vi "Forward Dynamics Demo.vi"() -> ()   [LabVIEW 2017, in "NI_Kinematics.lvlib"]
uses:
  <vilib>/robotics/Kinematics/NI_Kinematics.lvlib
panel:
  out "times":dbl[](array[numeric]) format="%#_40f"
  out "QD":dbl[][](array[numeric]) format="%#_6f"
  out "Q":dbl[][](array[numeric]) format="%#_6f"
  out "Time (ms)":u32
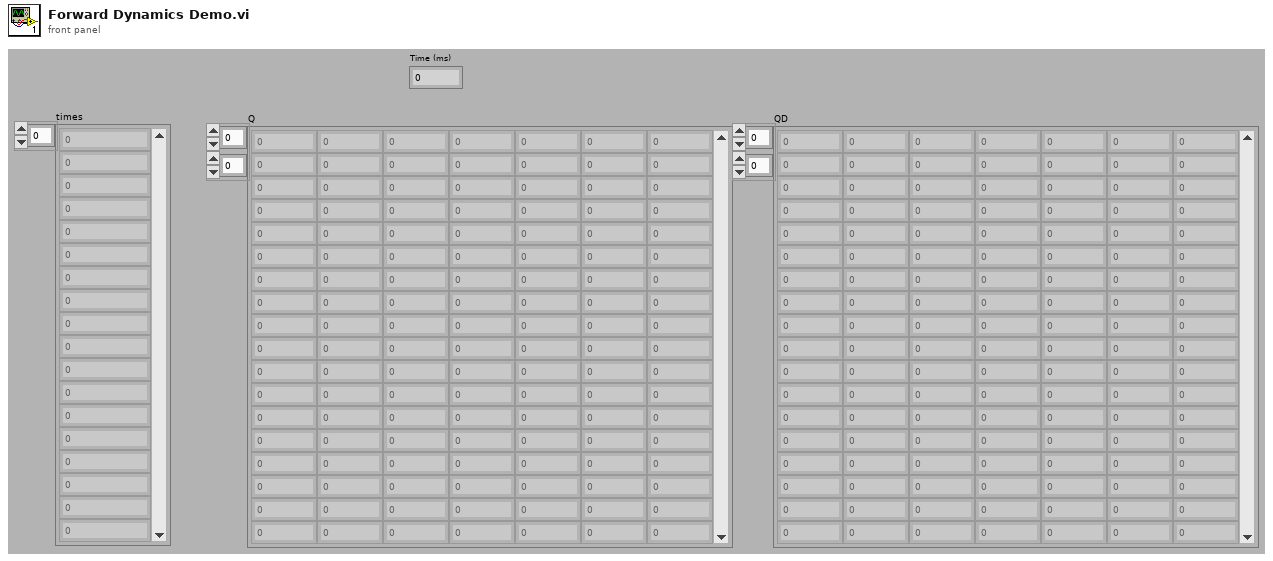
[diagram p1: front panel]
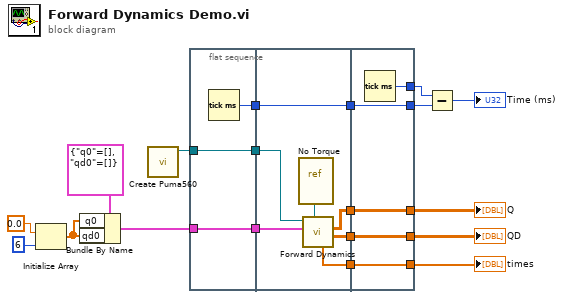
[diagram p0: block diagram]
diagram:
  n1 = Initialize Array(0.0 ("element"), 6 ("dimension size")) -> (w11:dbl[])
  n2 = Bundle By Name(cluster=cluster{"q0":dbl[], "qd0":dbl[]} {"q0"=[], "qd0"=[]} ("integration data"), "q0"=w11, "qd0"=w11) -> (w9:cluster{"q0":dbl[], "qd0":dbl[]})
  n3 = call <vilib>:"Create Puma560.vi"() -> ("Puma560 Robot"=w7:refnum<class "NI_Robotics_Serial Robot Arm.lvclass">)  [unwired: 1 in, 10 out]
  n4 = flat-sequence {
    tunnel: [w22] -> w19
    tunnel: w9 -> [w20]
    tunnel: w7 -> [w21]
    tunnel: [w21] -> w8
    tunnel: [w20] -> w1
    tunnel: w19 -> [w29]
    tunnel: [w29] -> w18
    tunnel: [w28] -> w17
    tunnel: w8 -> [w27]
    tunnel: [w26] -> w6
    tunnel: [w25] -> w3
    tunnel: w1 -> [w24]
    tunnel: [w33] -> w15
    tunnel: [w34] -> w5
    tunnel: w18 -> [w33]
    tunnel: [w32] -> w16
    tunnel: w17 -> [w34]
    tunnel: [w31] -> w4
    tunnel: w6 -> [w31]
    tunnel: [w30] -> w2
    tunnel: w3 -> [w30]
    frame #0 {
      n5 = Tick Count (ms)() -> (millisecond timer value=w22:u32)
    }
    frame #1 {
      n6 = vi-ref <vilib>:"No Torque.vi"() -> (w23:refnum<vi>)
      n7 = call <vilib>:"Forward Dynamics.vi"("torque function"=w23, "integration data"=w24, "serial arm in"=w27) -> ("joint velocity trajectory"=w28:dbl[][], "joint position trajectory"=w26:dbl[][], "times"=w25:dbl[])  [unwired: 4 in, 2 out]
    }
    frame #2 {
      n8 = Tick Count (ms)() -> (millisecond timer value=w32:u32)
    }
  }
  n9 = Subtract(x=w16, y=w15) -> (x-y=→"Time (ms)":u32)
  "Q" <- w4
  "QD" <- w5
  "times" <- w2
